vi "CallCameraSetup.vi"(8 "error in (no error)":errorcluster) -> (0 "error out":errorcluster)   [LabVIEW 2015, in "CameraSetup.lvlib"]
uses:
  CameraSetup.lvlib
  CameraSetup.vi
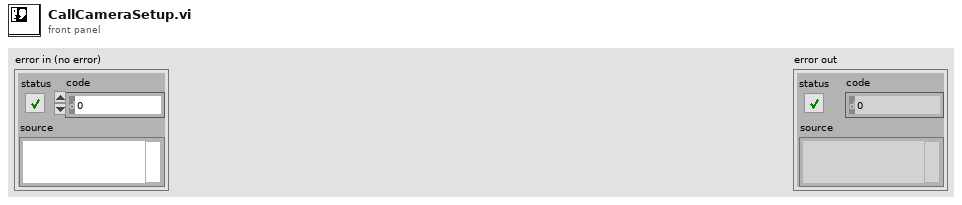
[diagram p1: front panel]
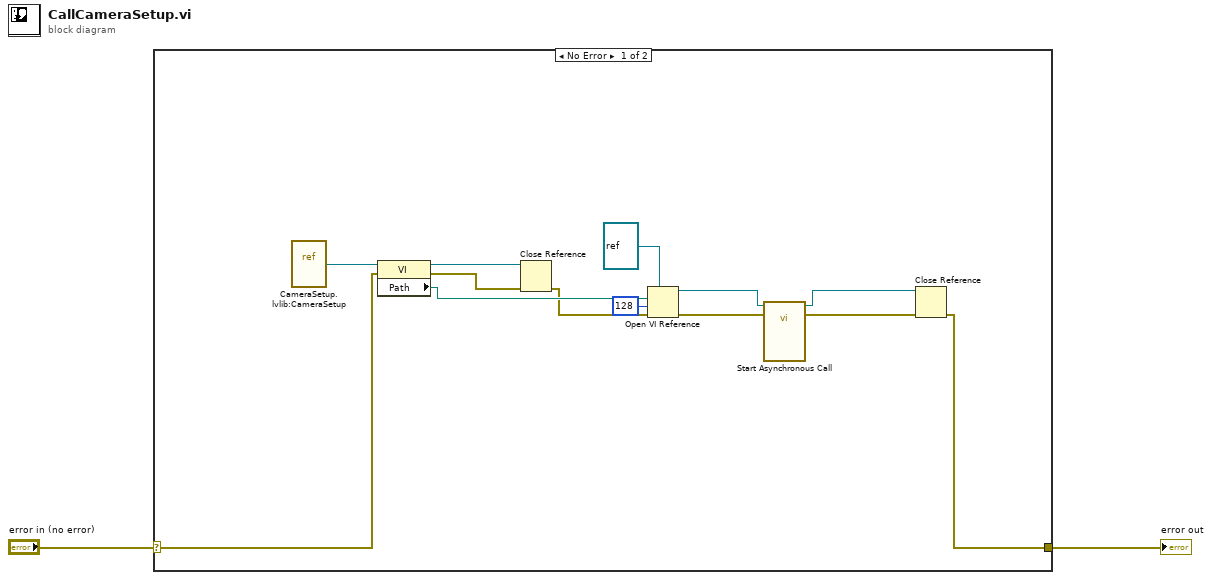
[diagram p0: block diagram]
diagram:
  n1 = case shown="No Error" "error in (no error)" {
    selector: "error in (no error)" -> [w5 w16]
    tunnel: [w4 w16] -> w1
    frame No Error {
      n2 = vi-ref "CameraSetup.lvlib:CameraSetup.vi"() -> (w15:refnum<vi>)
      n3 = property class="VI"(reference=w15, error in=w5) -> (reference out=w13:refnum<vi>, error out=w12:errorcluster, "Path"=w14:path)
      n4 = Close Reference(reference=w13, error in (no error)=w12) -> (error out=w11:errorcluster)
      n5 = Open VI Reference(type specifier VI Refnum (for type only)=refnum<vi> refnum, vi path=w14, options=128, error in (no error)=w11) -> (vi reference=w9:refnum<vi>, error out=w10:errorcluster)  [unwired: 2 in]
      n6 = call-by-ref "Start Asynchronous Call"(reference=w9, error in=w10) -> (reference out=w7:refnum<vi>, error out=w6:errorcluster)  [unwired: 12 in]
      n7 = Close Reference(reference=w7, error in (no error)=w6) -> (error out=w4:errorcluster)
    }
    frame Error {
    }
  }
  "error out" <- w1
